vi "Init Device.vi"(7 "Layout Ref":refnum<vi>, 8 "error in (no error)":errorcluster, 10 "Chan# Array":i32[](array[numeric]), 11 "SRS_SG380 in":refnum<class "SRS_SG380.lvclass">) -> (0 "error out":errorcluster, 3 "SRS_SG380 out":refnum<class "SRS_SG380.lvclass">)   [LabVIEW 2013, in "SRS_SG380.lvclass"]
doc: "Initialize the correct columns and their default appearance.\nUse the front panel to change default appearance of the device in the Add/Manage devices.\n\nOpen a specific device implementation for details."
uses:
  SRS_SG380.lvclass
  TypeDefs/ColumnAppearCluster.ctl
  ColumnVIs/SingleValCol/SingleValCol.lvclass
  ColumnVIs/Column/Column.lvclass
panel:
  in  "Amplitude Column Defaults":T1={"Column Name"="Amplitude", "Width"=30, "Bkgd"=[16448250], "Text"=[0]}
  in  "Freq Column Defaults":T1={"Column Name"="Frequency", "Width"=30, "Bkgd"=[16448250], "Text"=[0]}
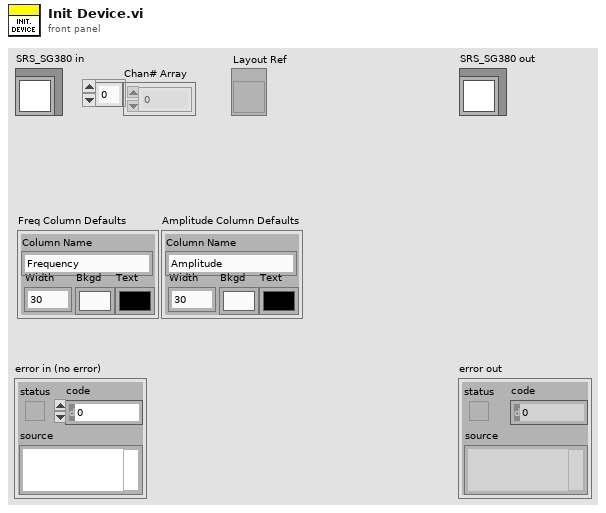
[diagram p1: front panel]
types:
  T1 = typedef "ColumnAppearCluster.ctl" = cluster{"Column Name":string, "Width":u32, "Bkgd":u32[], "Text":u32[]}
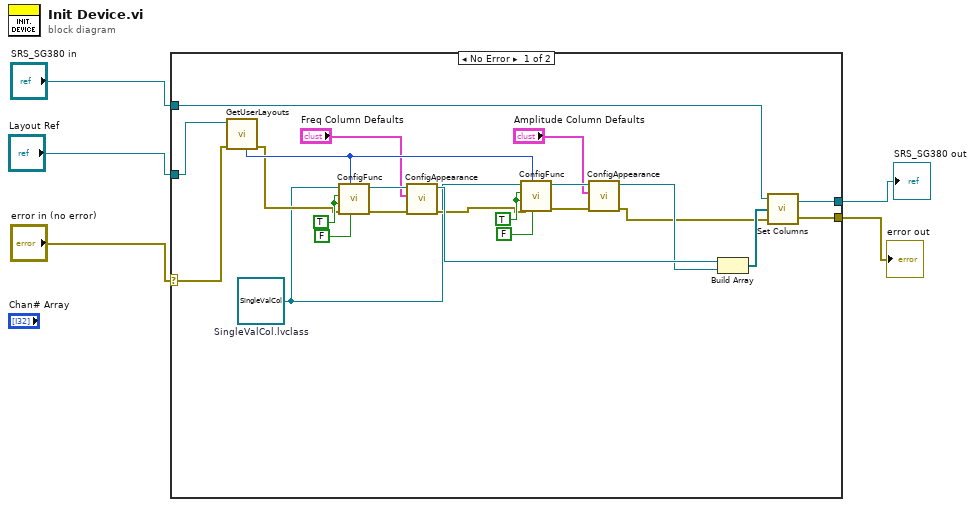
[diagram p0: block diagram]
diagram:
  n1 = case shown="No Error" "error in (no error)" {
    selector: "error in (no error)" -> [w27 w29]
    tunnel: "SRS_SG380 in" -> [w18 w30]
    tunnel: [w17 w30] -> w2
    tunnel: [w12 w29] -> w3
    tunnel: "Layout Ref" -> [w28 _]
    frame No Error {
      w23 = TRUE ("Disableable? (True)")
      w25 = TRUE ("Disableable? (True)")
      w9 = refnum<class "SingleValCol.lvclass"> refnum  # SingleValCol.lvclass
      n2 = call "GetUserLayouts.vi"("error in (no error)"=w27, "Layout Ring Refnum"=w28) -> ("error out"=w16:errorcluster, "Num User Layouts"=w22:i32)  [unwired: 5 in, 3 out]
      n3 = call "ConfigFunc.vi"("isRampable? (True"=FALSE, "Num Layouts (ignored)"=w22, "error in (no error)"=w16, "isVariable? (True)"=w25, "Disableable? (True)"=w25, "Column in"=w9) -> ("error out"=w15:errorcluster, "Column out"=w26:refnum<class "SingleValCol.lvclass">)  [unwired: 4 in]
      n4 = call "ConfigAppearance.vi"("error in (no error)"=w15, "Column Appearance"="Freq Column Defaults", "Column in"=w26) -> ("error out"=w14:errorcluster, "Column out"=w21:refnum<class "SingleValCol.lvclass">)  [unwired: 7 in]
      n5 = call "ConfigFunc.vi"("isRampable? (True"=FALSE, "Num Layouts (ignored)"=w22, "error in (no error)"=w14, "isVariable? (True)"=w23, "Disableable? (True)"=w23, "Column in"=w9) -> ("error out"=w13:errorcluster, "Column out"=w24:refnum<class "SingleValCol.lvclass">)  [unwired: 4 in]
      n6 = call "ConfigAppearance.vi"("error in (no error)"=w13, "Column Appearance"="Amplitude Column Defaults", "Column in"=w24) -> ("error out"=w6:errorcluster, "Column out"=w20:refnum<class "SingleValCol.lvclass">)  [unwired: 7 in]
      n7 = Build Array(w21, w20) -> (w19:refnum<class "SingleValCol.lvclass">[])
      n8 = call-dynamic "Set Columns.vi"("error in (no error)"=w6, "Columns"=w19, "Device in"=w18) -> ("error out"=w12:errorcluster, "Device out"=w17:refnum<class "SRS_SG380.lvclass">)  [unwired: 1 in]
    }
    frame Error {
    }
  }
  "error out" <- w3
  "SRS_SG380 out" <- w2
